vi "Inicio_ALL.vi"(7 "Error In":errorcluster) -> (20 "Turbi_IN out":refnum<k21>, 21 "UV_Lamp out":refnum<k21>, 22 "V_Bombas out":refnum<k21>, 23 "Bombas_OUT out":refnum<k21>, 24 "Bombas_IN out":refnum<k21>, 27 "error out":errorcluster)   [LabVIEW 2013]
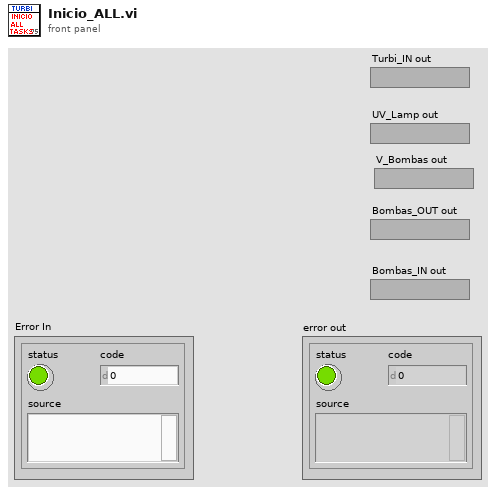
[diagram p1: front panel]
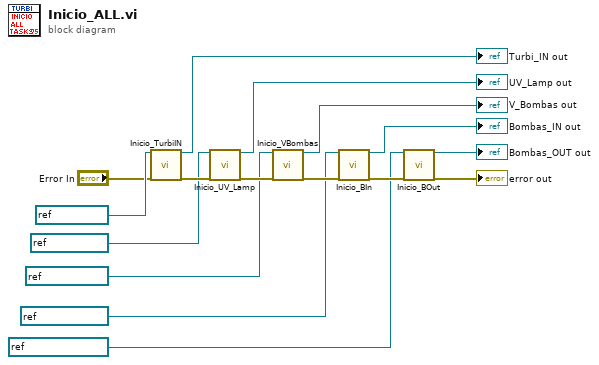
[diagram p0: block diagram]
diagram:
  n1 = call "Inicio_TurbiIN.vi"("task/channels in"=refnum<k21> "Turbi_IN", "error in"="Error In") -> ("Refnum out"=→"Turbi_IN out":refnum<k21>, "error out"=w4:errorcluster)  [unwired: 16 in]
  n2 = call "Inicio_UV_Lamp.vi"("Refnum in"=refnum<k21> "UV_Lamp" ("task/channels in"), "error in (no error)"=w4) -> ("task out"=→"UV_Lamp out":refnum<k21>, "error out"=w6:errorcluster)  [unwired: 16 in]
  n3 = call "Inicio_VBombas.vi"("Refnum in"=refnum<k21> "V_Bombas" ("task/channels in"), "error in (no error)"=w6) -> ("Refnum out"=→"V_Bombas out":refnum<k21>, "error out"=w9:errorcluster)  [unwired: 16 in]
  n4 = call "Inicio_BIn.vi"("Refnum in"=refnum<k21> "Bombas_IN", "error in (no error)"=w9) -> ("Refnum out"=→"Bombas_IN out":refnum<k21>, "error out"=w10:errorcluster)  [unwired: 16 in]
  n5 = call "Inicio_BOut.vi"("Refnum in"=refnum<k21> "Bombas_OUT", "error in (no error)"=w10) -> ("Refnum out"=→"Bombas_OUT out":refnum<k21>, "error out"=→"error out":errorcluster)  [unwired: 16 in]
